vi "Get OFDM Channel EVM.vi"(8 "error in (no error)":errorcluster, 11 "niDTS WLAN INSTR TX in":refnum<class "niDTS WLAN INSTR TX.lvclass">) -> (0 "error out":errorcluster, 2 "OFDM Channel EVM":T1, 3 "niDTS WLAN INSTR TX out":refnum<class "niDTS WLAN INSTR TX.lvclass">)   [LabVIEW 2015, in "niDTS WLAN.lvlib" / "niDTS WLAN INSTR TX.lvclass"]
uses:
  niDTS WLAN INSTR TX.lvclass
  Tests/Tx Test/Includes/niDTS WLAN Tx Test INC MOD EVM Results.ctl
  Tests/Tx Test/Includes/Results/niDTS Tx RES INC EVM.ctl
  niDTS WLAN INSTR TX.lvclass/niDTS WLAN INSTR TX.ctl
  RiviInstDriver/niRfsaWlan/Objects/niRfsaWlan.lvclass
  niDTS WLAN.lvlib
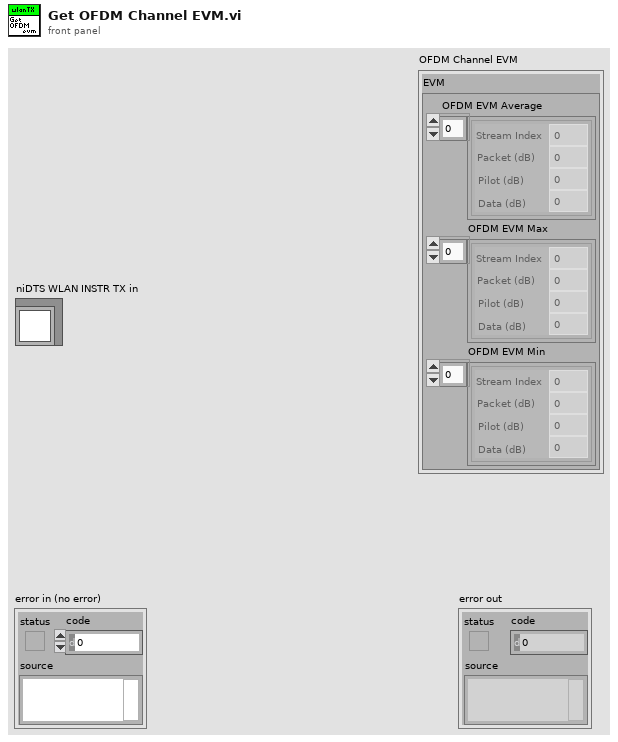
[diagram p1: front panel]
types:
  T1 = typedef "niDTS WLAN.lvlib/niDTS WLAN Tx Test INC MOD EVM Results.ctl" = cluster{"EVM":cluster{"OFDM EVM Average":T2[], "OFDM EVM Max":T2[], "OFDM EVM Min":T2[]}}
  T2 = typedef "niDTS WLAN.lvlib/niDTS Tx RES INC EVM.ctl" = cluster{"Stream Index":i32, "Packet (dB)":dbl, "Pilot (dB)":dbl, "Data (dB)":dbl}
  T3 = typedef "niRfsaWlan.lvclass/niRfsaWlan INC Handle.ctl" = refnum<data-value>
  T4 = typedef "niDTS WLAN.lvlib/niDTS WLAN Tx Test INC Parameters.ctl" = cluster{"Standard":T5, "DSSS Data Rate (Mbps)":T6, "OFDM Data Rate (Mbps)":T7, "MCS Index":i32, "N spatial streams":i32, "Chains":bool[], "BandWidth (Hz)":T8, "Channel":i32, "Gard Interval":T9, "FEC Coding":T10, "Dut Tx Power":dbl, "16 symbols":bool, "payload length bytes":i32, "idle interval":dbl, "External Attenuation":dbl[], "Acquisition Parameters ":T11, "TXP Measurement Parameters":T12, "ModAcc Measurement Paramaters":T13, "ModAcc DSSS Paramaters":T14, "SEM Measurement Parameters":T16, "OBW Measurement Parameters":T17, "DSSS Power Ramp":T18, "Enable Traces":bool}
  T5 = typedef "niDTS WLAN.lvlib/niDTS WLAN INC Standard.ctl" = enum16{"802.11 b DSSS", "802.11 a/g OFDM", "802.11 n HT", "802.11 ac VHT"}
  T6 = typedef "niDTS WLAN.lvlib/niDTS WLAN INC DSSS Data Rate.ctl" = enum16{"1", "2", "5.5", "11"}
  T7 = typedef "niDTS WLAN.lvlib/niDTS WLAN INC OFDM Data Rate.ctl" = enum16{"6", "9", "12", "18", "24", "36", "48", "54"}
  T8 = typedef "niDTS WLAN.lvlib/niDTS WLAN INC CH BW.ctl" = enum16{"20 MHz", "40 MHz", "80 MHz", "160 MHz"}
  T9 = typedef "niDTS WLAN.lvlib/niDTS WLAN INC GI.ctl" = enum16{"LONG", "SHORT"}
  T10 = typedef "niDTS WLAN.lvlib/niDTS WLAN INC FEC Coding.ctl" = enum16{"BCC", "LDPC"}
  T11 = typedef "niDTS WLAN.lvlib/niDTS WLAN DUT INC Acquisition Parameters.ctl" = cluster{"Acquisition Length Mode":enum16{"AUTO", "MANUAL"}, "Acquisition Length (s)":dbl, "Auto Level":bool}
  T12 = typedef "niDTS WLAN.lvlib/niDTS WLAN INC TXP Measurement Parameters.ctl" = cluster{"TXP Power Enable":bool, "TXP Averages":i32}
  T13 = typedef "niDTS WLAN.lvlib/niDTS WLAN INC ModAcc Measurement Parameters.ctl" = cluster{"ModAcc Enable":bool, "Header Detection":enum16{"MANUAL", "FIRST", "ALL"}, "Averages":i32, "Amplitude Tracking":bool, "Channel Tracking":bool, "Time Tracking":bool, "Phase Tracking":enum16{"NONE", "STANDARD", "CSF", "INSTANT"}, "Clock Offset Est":bool, "Impairments Est":bool, "CFO Estimation":enum16{"PAMBLE", "PDATA"}}
  T14 = typedef "niDTS WLAN.lvlib/niDTS WLAN INC DSSS ModAcc Measurement Parameters.ctl" = cluster{"DC Offset Compensation":bool, "Equalization":bool, "Phase Tracking":bool, "Chip Start Location":i16, "Max Chips Used":i16, "Pulse Shaping FilterType":T15, "Pulse Shaping Filter Coefficient":dbl}
  T15 = typedef "niDTS WLAN.lvlib/niDTS WLAN INC Pulse Shaping Filter Type.ctl" = enum16{"NONE", "RCOSINE", "RRCOSINE", "GAUSSIAN"}
  T16 = typedef "niDTS WLAN.lvlib/niDTS WLAN INC SEM Measurement Parameters.ctl" = cluster{"SEM Enable":bool, "SEM Averages":i32, "Auto Span Enable":bool, "Frequency Span (Hz)":dbl, "Measurement Type":enum16{"Standard", "Legacy", "Custom"}, "Mask Frequencies (Hz)":dbl[], "Mask Power Offsets (dB)":dbl[]}
  T17 = typedef "niDTS WLAN.lvlib/niDTS WLAN INC OBW Measurement Parameters.ctl" = cluster{"OBW Enable":bool, "OBW Averages":i32}
  T18 = typedef "niDTS WLAN.lvlib/niDTS WLAN INC DSSS Power Ramp Parameters.ctl" = cluster{"Power Ramp Enable":bool, "Averages":i32, "Thresholds":cluster{"Up Low (%)":dbl, "Down Low (%)":dbl, "Up High (%)":dbl, "Down High (%)":dbl}}
  T19 = cluster{"ChannelIndex":i32, "RmsEvm":dbl, "RmsPilotEvm":dbl, "RmsDataEvm":dbl}[]
  T20 = cluster{"ChannelIndex":i32, "RmsEvm":dbl, "RmsPilotEvm":dbl, "RmsDataEvm":dbl}
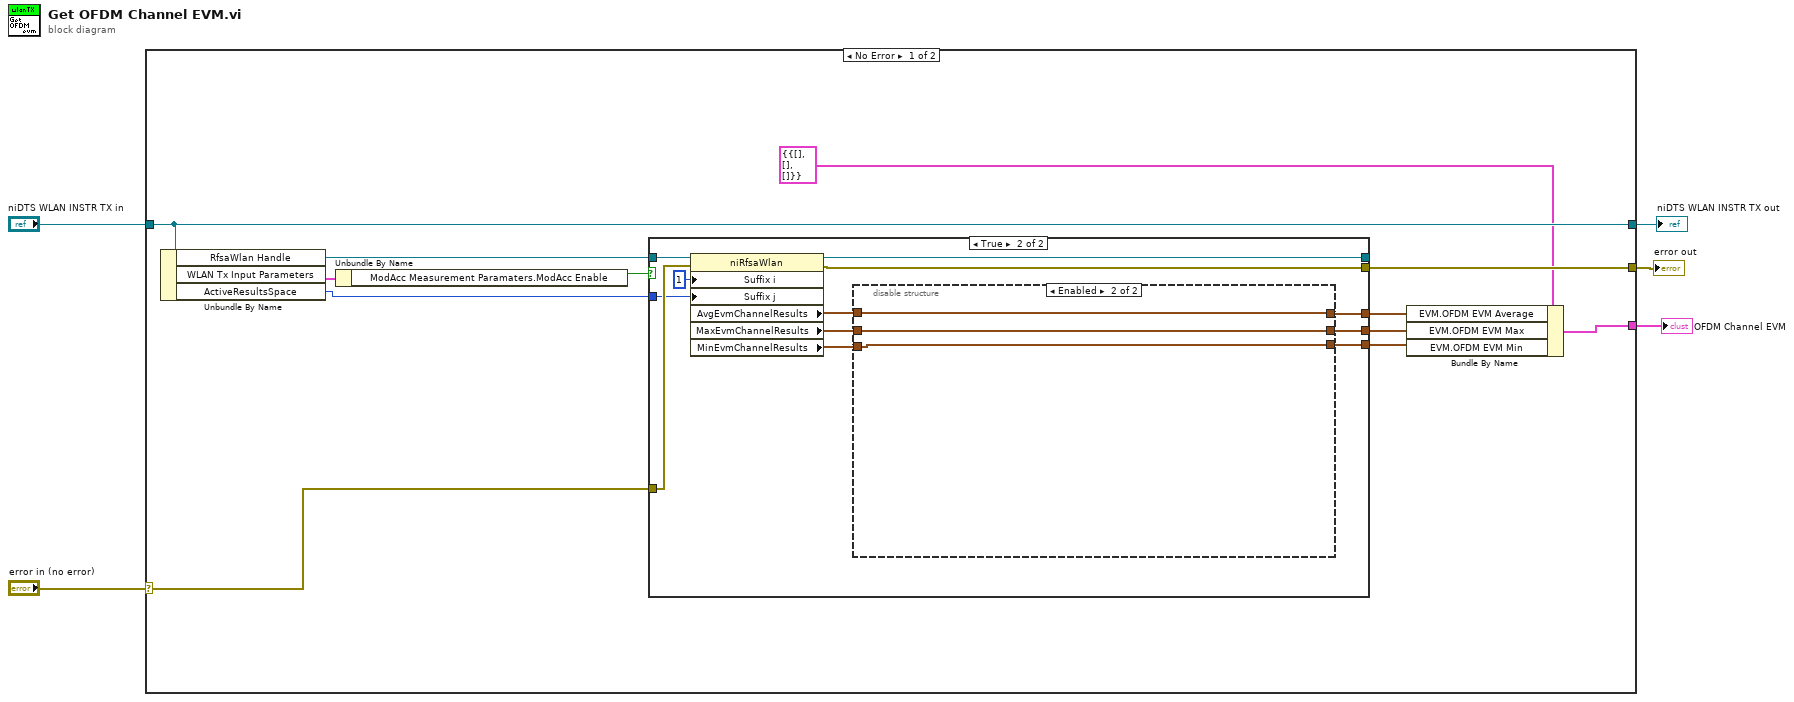
[diagram p0: block diagram]
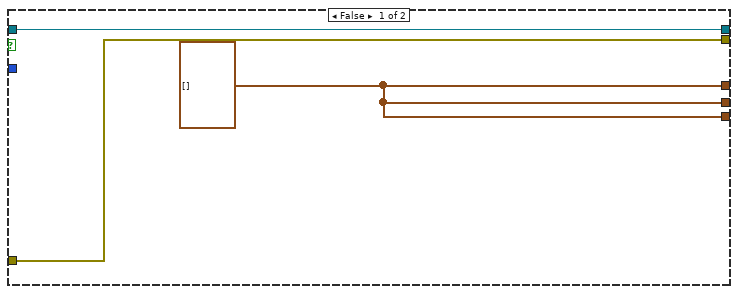
[diagram p2: hidden frame]
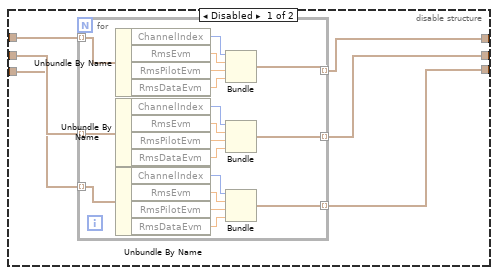
[diagram p3: hidden frame]
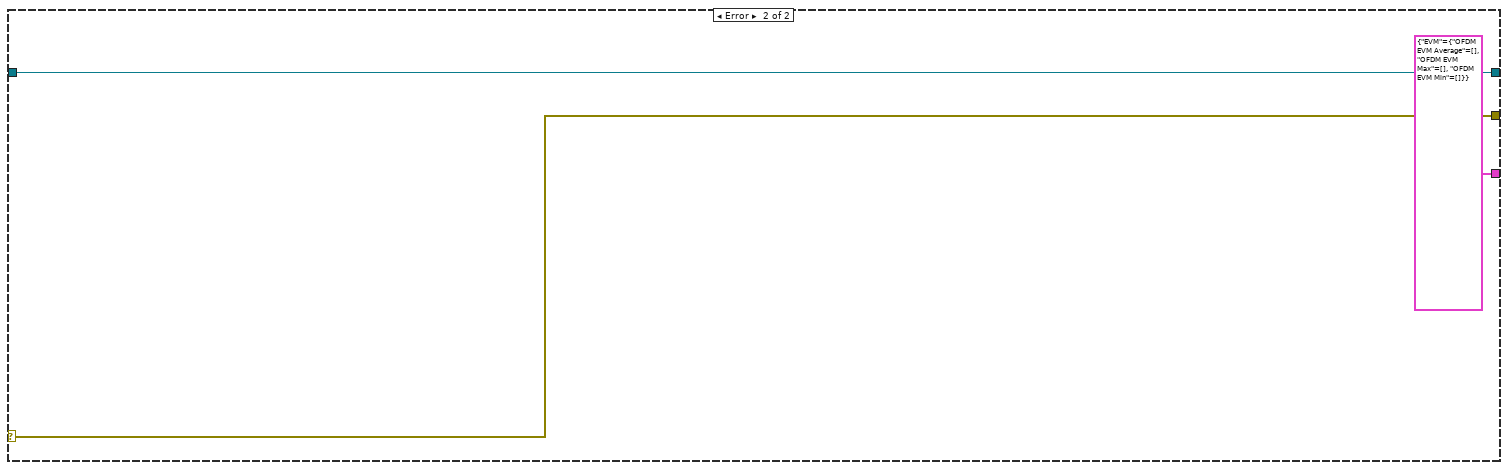
[diagram p4: hidden frame]
diagram:
  n1 = case shown="No Error" "error in (no error)" {
    selector: "error in (no error)" -> [w15 w62]
    tunnel: [w12 w62] -> w4
    tunnel: [w17 w61] -> w2
    tunnel: "niDTS WLAN INSTR TX in" -> [w17 w61]
    tunnel: [w7 T1 {"EVM"={"OFDM EVM Average"=[], "OFDM EVM Max"=[], "OFDM EVM Min"=[]}} ("OFDM Stream EVM 2")] -> w1
    frame No Error {
      n2 = Unbundle By Name(w17) -> ("RfsaWlan Handle"=w13:T3, "WLAN Tx Input Parameters"=w16:T4, "ActiveResultsSpace"=w6:u8)
      n3 = Unbundle By Name(w16) -> ("ModAcc Measurement Paramaters.ModAcc Enable"=w14:bool)
      n4 = case shown="True" w14 {
        tunnel: w15 -> [w19 w30]
        tunnel: w13 -> [w20 w31]
        tunnel: [w20 w29] -> _
        tunnel: [w18 w24] -> w10
        tunnel: [w19 w28] -> w12
        tunnel: [w18 w23] -> w9
        tunnel: [w18 w22] -> w8
        tunnel: w6 -> [_ w21]
        frame False {
          w18 = T19 [] ("AvgEvmStreamResults[]")
        }
        frame True {
          n5 = property class="niRfsaWlan"(reference=w31, error in=w30, "Suffix i"=1 ("Active Channel:Result Space"), "Suffix j"=w21) -> (reference out=w29:T3, error out=w28:errorcluster, "AvgEvmChannelResults"=w27:T19, "MaxEvmChannelResults"=w26:T19, "MinEvmChannelResults"=w25:T19)
          n6 = disable-structure shown="Enabled" {
            disable-tunnel: w27 -> [w38 w59]
            disable-tunnel: w26 -> [w37 w58]
            disable-tunnel: w25 -> [w36 w57]
            disable-tunnel: [w35 w59] -> w24
            disable-tunnel: [w34 w58] -> w23
            disable-tunnel: [w33 w57] -> w22
            frame Disabled {
              n7 = for {
                tunnel: w38 -> [w56] mode=indexing
                tunnel: w37 -> [w51] mode=indexing
                tunnel: w36 -> [w42] mode=indexing
                tunnel: [w41] -> w35 mode=indexing
                tunnel: [w40] -> w34 mode=indexing
                tunnel: [w39] -> w33 mode=indexing
                n8 = Unbundle By Name(w56) -> ("ChannelIndex"=w55:i32, "RmsEvm"=w54:dbl, "RmsPilotEvm"=w53:dbl, "RmsDataEvm"=w52:dbl)
                n9 = Unbundle By Name(w51) -> ("ChannelIndex"=w50:i32, "RmsEvm"=w49:dbl, "RmsPilotEvm"=w48:dbl, "RmsDataEvm"=w47:dbl)
                n10 = Unbundle By Name(w42) -> ("ChannelIndex"=w43:i32, "RmsEvm"=w44:dbl, "RmsPilotEvm"=w45:dbl, "RmsDataEvm"=w46:dbl)
                n11 = Bundle("ChannelIndex"=w55, "RmsEvm"=w54, "RmsPilotEvm"=w53, "RmsDataEvm"=w52) -> (w41:T20)  [unwired: 1 in]
                n12 = Bundle("ChannelIndex"=w50, "RmsEvm"=w49, "RmsPilotEvm"=w48, "RmsDataEvm"=w47) -> (w40:T20)  [unwired: 1 in]
                n13 = Bundle("ChannelIndex"=w43, "RmsEvm"=w44, "RmsPilotEvm"=w45, "RmsDataEvm"=w46) -> (w39:T20)  [unwired: 1 in]
              }
            }
            frame Enabled {
            }
          }
        }
      }
      n14 = Bundle By Name(cluster=T1 {"EVM"={"OFDM EVM Average"=[], "OFDM EVM Max"=[], "OFDM EVM Min"=[]}} ("OFDM Stream EVM 2"), "EVM.OFDM EVM Average"=w10, "EVM.OFDM EVM Max"=w9, "EVM.OFDM EVM Min"=w8) -> (w7:T1)
    }
    frame Error {
    }
  }
  "error out" <- w4
  "niDTS WLAN INSTR TX out" <- w2
  "OFDM Channel EVM" <- w1
